vi "Get_Analog_Value.vi"(7 "error in":errorcluster, 9 "Samples qty":i32, 10 "Device Session In":refnum<visa-resource-name>) -> (0 "error out":errorcluster, 2 "Output values":i32[](array[numeric]), 3 "Device Session Out":refnum<visa-resource-name>)   [LabVIEW 2017]
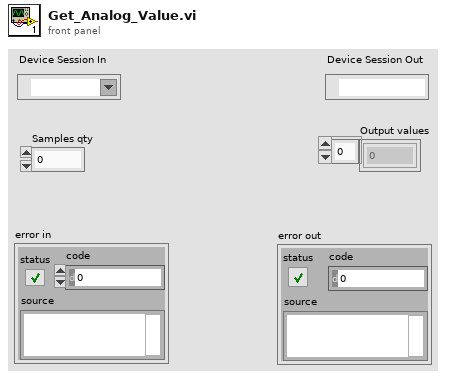
[diagram p1: front panel]
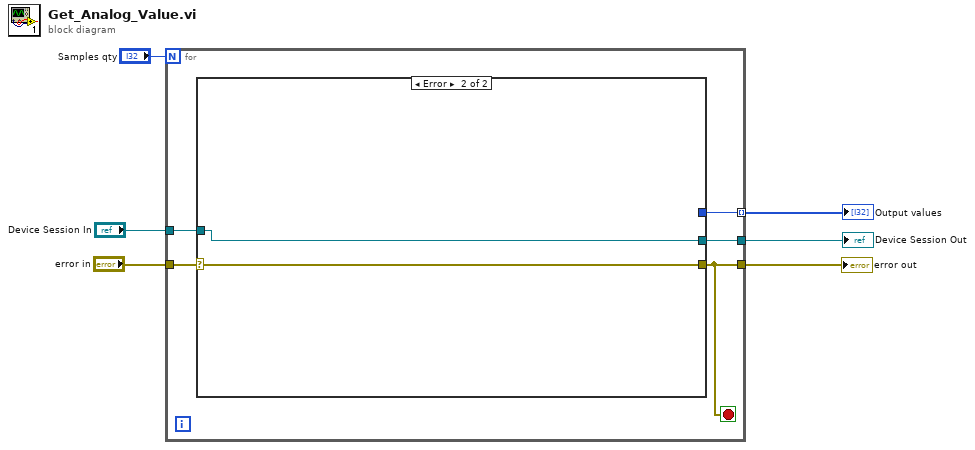
[diagram p0: block diagram]
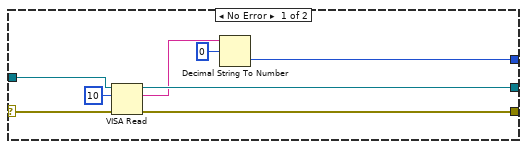
[diagram p2: hidden frame]
diagram:
  n1 = for {
    N: "Samples qty" -> [_]
    tunnel: [w11] -> w6
    tunnel: [w7] -> w5
    tunnel: [w10] -> w4 mode=indexing
    tunnel: "Device Session In" -> [w9]
    tunnel: "error in" -> [w8]
    stop <- w7 stop-if-true
    n2 = case shown="Error" w8 {
      selector: w8 -> [w14 w21]
      tunnel: [w19 w21] -> w7
      tunnel: [w18 w20] -> w11
      tunnel: [w13 _] -> w10
      tunnel: w9 -> [w12 w20]
      frame No Error {
        n3 = VISA Read(VISA resource name=w12, byte count=u32 10, error in (no error)=w14) -> (VISA resource name out=w18:refnum<visa-resource-name>, read buffer=w17:string, error out=w19:errorcluster)  [unwired: 1 out]
        n4 = Decimal String To Number(string=w17, offset=0 ("offset (0)")) -> (number=w13:i32)  [unwired: 1 in, 1 out]
      }
      frame Error {
      }
    }
  }
  "Device Session Out" <- w6
  "error out" <- w5
  "Output values" <- w4
